vi "Get Service Name.vi"(8 "error in (no error)":errorcluster) -> (0 "error out":errorcluster, 3 "Service Name":string)   [LabVIEW 2015, in "CLI.lvclass"]
uses:
  CLI.lvclass
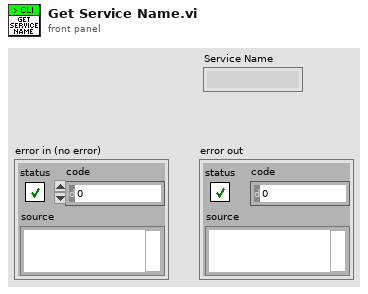
[diagram p1: front panel]
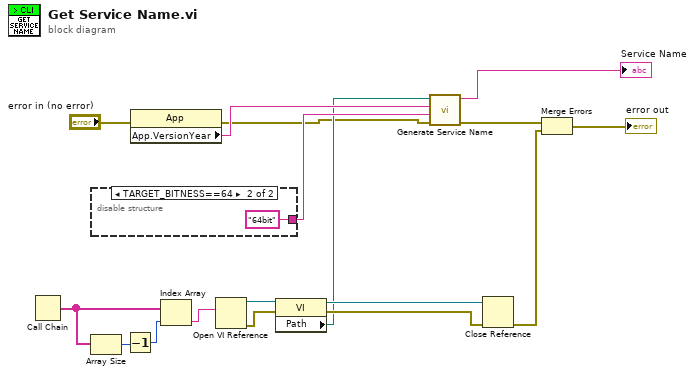
[diagram p0: block diagram]
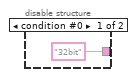
[diagram p2: hidden frame]
diagram:
  n1 = Call Chain() -> (call chain=w14:string[])
  n2 = Array Size(array=w14) -> (size(s)=w16:i32)
  n3 = disable-structure shown="TARGET_BITNESS==64" {
    disable-tunnel: ["32bit" "64bit"] -> w7
    frame condition #0 {
    }
    frame condition #1 (active) {
    }
  }
  n4 = Decrement(x=w16) -> (x-1=w15:i32)
  n5 = property class="App"(error in="error in (no error)") -> (error out=w4:errorcluster, "App.VersionYear"=w8:string)  [unwired: 1 in, 1 out]
  n6 = Index Array(array=w14, index=w15) -> (element=w13:string)
  n7 = Open VI Reference(vi path=w13) -> (vi reference=w12:refnum<vi>, error out=w11:errorcluster)  [unwired: 5 in]
  n8 = property class="VI"(reference=w12, error in=w11) -> (reference out=w9:refnum<vi>, error out=w10:errorcluster, "Path"=w6:path)
  n9 = call "Generate Service Name.vi"("error in (no error)"=w4, "Bitness Text"=w7, "LV Version"=w8, "VI Path"=w6) -> ("error out"=w3:errorcluster, "Service Name"=→"Service Name":string)  [unwired: 6 in]
  n10 = Close Reference(reference=w9, error in (no error)=w10) -> (error out=w1:errorcluster)
  n11 = Merge Errors(w3, w1) -> (→"error out":errorcluster)
